vi "Y5140_RdPower.vi"(8 "error in (no error)":errorcluster caption="错误输入（无错误）", 11 "Index":u32) -> (0 "error out":errorcluster caption="错误输出", 1 "T/F":bool, 2 "Value":sgl)   [LabVIEW 2015]
uses:
  <vilib>/Instr/_visa.llb/VISA Configure Serial Port (Instr).vi
panel:
  in  "MyIndex":u8
  out "VISA":refnum<visa-resource-name> caption="VISA资源名称输出"
  out "Rx":string
  out "Tx":string
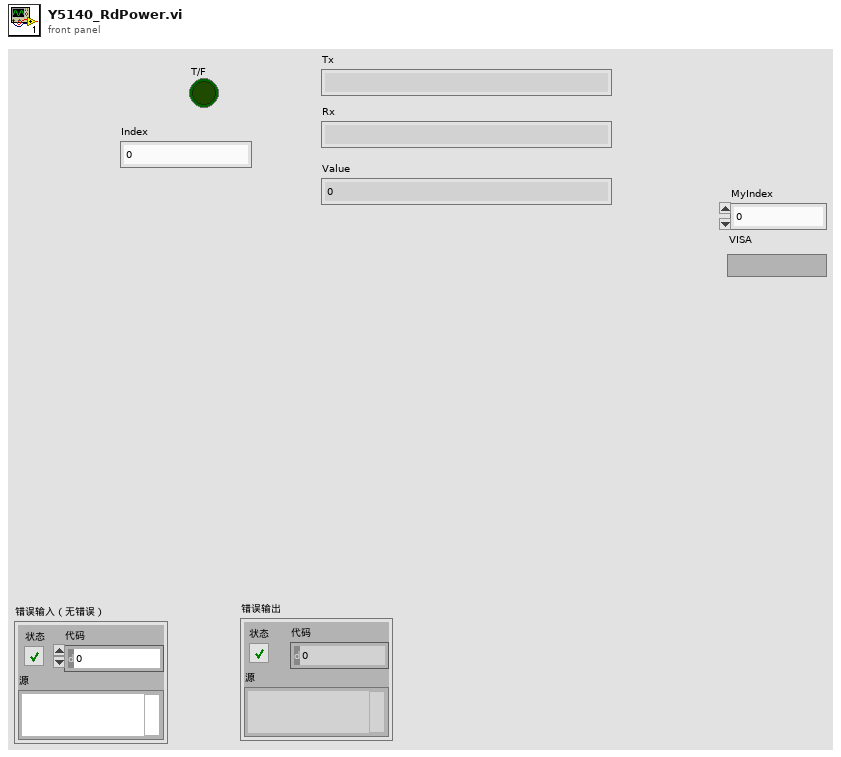
[diagram p1: front panel]
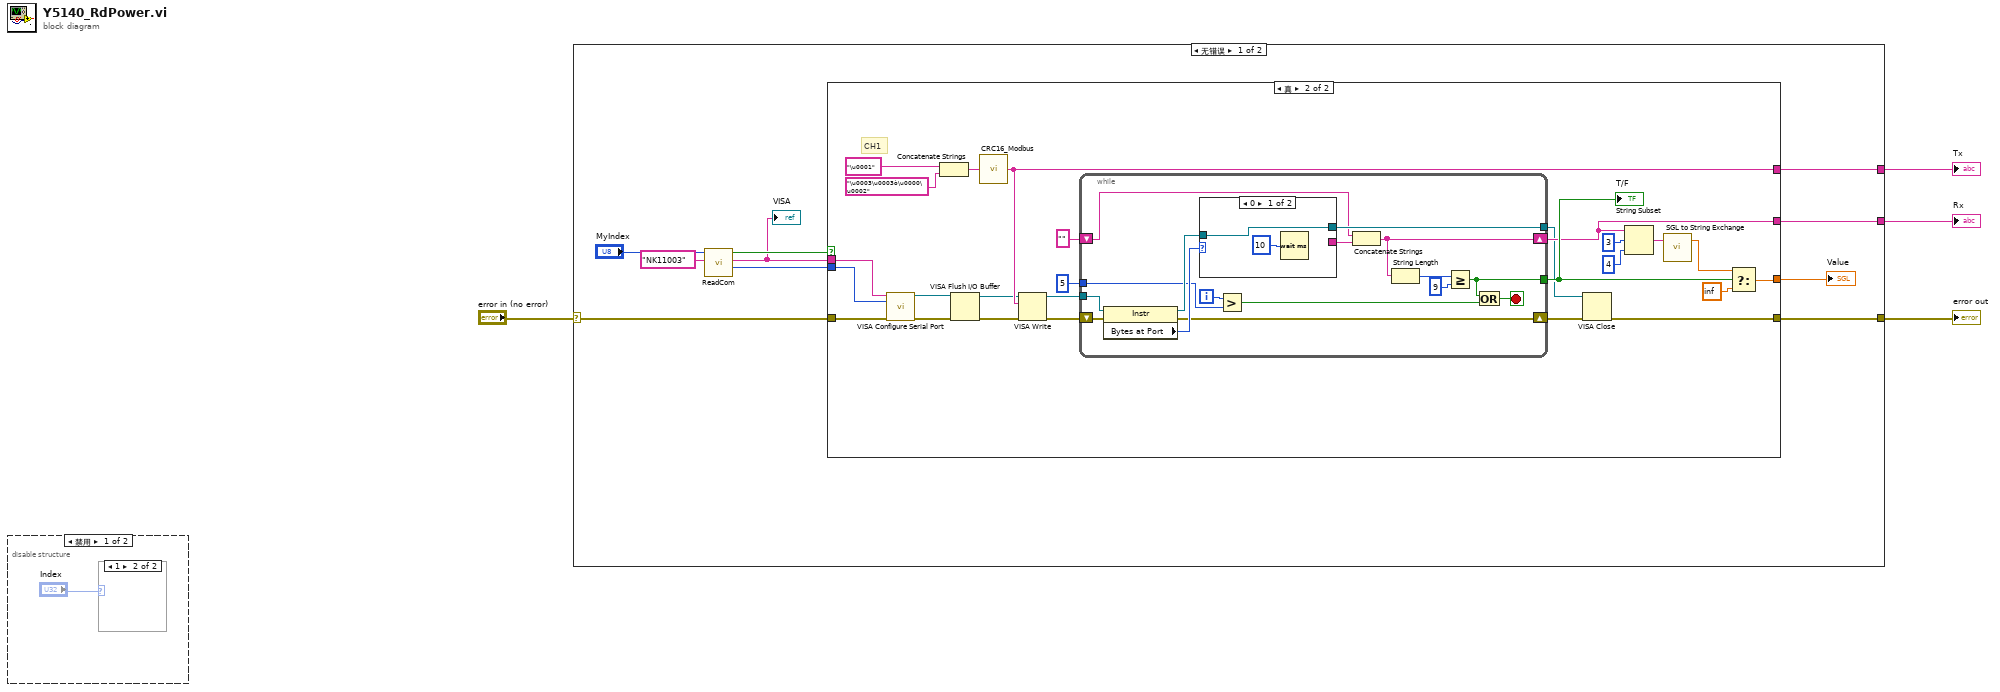
[diagram p0: block diagram]
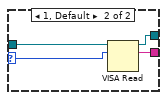
[diagram p5: hidden frame]
diagram:
  n1 = disable-structure shown="禁用" {
    frame Disabled {
      n2 = case shown="1" "Index" {
        frame 0, Default {
        }
        frame 1 {
        }
      }
    }
    frame Enabled {
    }
  }
  n3 = case shown="无错误" "error in (no error)" {
    selector: "error in (no error)" -> [w14 w64]
    tunnel: [w13 w64] -> w3
    tunnel: [w12 _] -> w2
    tunnel: [w11 _] -> w1
    frame No Error {
      n4 = call "ReadCom.vi"("仪器名称"="NK11003", "MyIndex"="MyIndex") -> ("Baudrate"=w6:i32, "COM"=w7:string, "OK?"=w8:bool)  [unwired: 7 in]
      "VISA" <- w7
      n5 = case shown="真" w8 {
        tunnel: [_ w40] -> w15
        tunnel: w14 -> [_ w39]
        tunnel: [_ w17] -> w13
        tunnel: [_ w37] -> w12
        tunnel: [_ w36] -> w11
        tunnel: w7 -> [_ w20]
        tunnel: w6 -> [_ w19]
        frame False {
        }
        frame True {
          # "CH1"
          n6 = call-poly "VISA Configure Serial Port"("VISA resource name"=w20, "baud rate (9600)"=w19, "error in (no error)"=w39) -> ("VISA resource name out"=w18:refnum<visa-resource-name>, "error out"=w21:errorcluster)  [unwired: 11 in]
          n7 = Concatenate Strings("\u0001", "\u0003\u0003ò\u0000\u0002") -> (w23:string)
          n8 = VISA Flush I/O Buffer(VISA resource name=w18, error in (no error)=w21) -> (VISA resource name out=w35:refnum<visa-resource-name>, error out=w34:errorcluster)  [unwired: 1 in]
          n9 = call "CRC16_Modbus.vi"("需要校验的数据"=w23) -> ("String+CRC16"=w37:string)
          n10 = VISA Write(VISA resource name=w35, write buffer=w37, error in (no error)=w34) -> (VISA resource name out=w33:refnum<visa-resource-name>, error out=w32:errorcluster)  [unwired: 1 out]
          n11 = while {
            tunnel: w33 -> [w57]
            tunnel: [w54] -> w16
            shift-right: [w46] -> w36
            shift-left: "" -> [w52]
            tunnel: 5 ("y") -> [w50]
            tunnel: [w42] -> w41
            shift-right: [w48] -> w38
            shift-left: w32 -> [w49]
            i -> [w51]
            stop <- w43 stop-if-true
            n12 = property class="Instr"(reference=w57, error in=w49) -> (reference out=w55:refnum<visa-resource-name>, error out=w48:errorcluster, "Bytes at Port"=w56:u32)
            n13 = case shown="0" w56 {
              selector: w56 -> [_ w62]
              tunnel: w55 -> [w59 w63]
              tunnel: [w59 w61] -> w54
              tunnel: [_ w60] -> w53
              frame 0 {
                n14 = Wait (ms)(milliseconds to wait=u32 10 ("等待时间（毫秒）")) -> ()  [unwired: 1 out]
              }
              frame 1, Default {
                n15 = VISA Read(VISA resource name=w63, byte count=w62) -> (VISA resource name out=w61:refnum<visa-resource-name>, read buffer=w60:string)  [unwired: 1 in, 2 out]
              }
            }
            n16 = Greater?(x=w51, y=w50) -> (0:w47:bool)
            n17 = Concatenate Strings(w52, w53) -> (w46:string)
            n18 = String Length(string=w46) -> (length=w45:i32)
            n19 = Greater Or Equal?(x=w45, y=9) -> (x >= y?=w42:bool)
            n20 = Or(x=w42, y=w47) -> (x .or. y?=w43:bool)
          }
          "T/F" <- w41
          n21 = VISA Close(VISA resource name=w16, error in (no error)=w38) -> (error out=w17:errorcluster)
          n22 = String Subset(string=w36, offset (0)=3 ("偏移量(0)"), length (rest)=4 ("长度（剩余）")) -> (substring=w27:string)
          n23 = call "SGL to String Exchange.vi"("4字节字符串"=w27) -> ("IEE754Floatout"=w26:sgl)  [unwired: 1 in, 1 out]
          n24 = Select(t=w26, s=w41, f=sgl inf) -> (s? t:f=w40:sgl)
        }
      }
      "Value" <- w15
    }
    frame Error {
    }
  }
  "error out" <- w3
  "Tx" <- w2
  "Rx" <- w1
